vi "readI64.vi"(8 "error in (no error)":errorcluster, 11 "ModbusBuffer in":refnum<class "ModbusBuffer.lvclass">) -> (0 "error out":errorcluster, 2 "Output":i64, 3 "ModbusBuffer out":refnum<class "ModbusBuffer.lvclass">)   [LabVIEW 2016, in "RTModbus.lvlib" / "ModbusBuffer.lvclass"]
uses:
  ModbusBuffer.lvclass
  ModbusBuffer.lvclass/ModbusBuffer.ctl
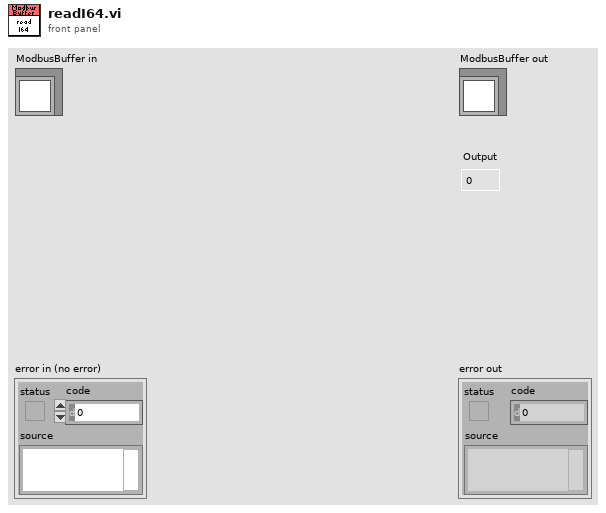
[diagram p1: front panel]
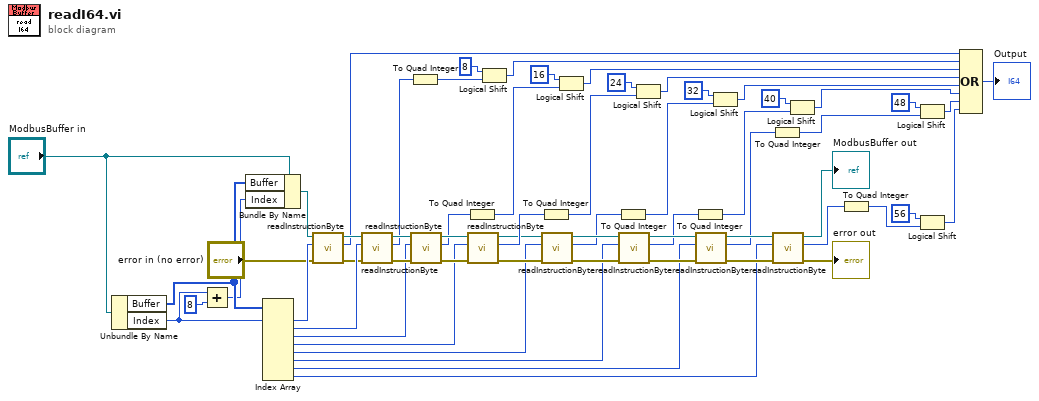
[diagram p0: block diagram]
diagram:
  n1 = Unbundle By Name("ModbusBuffer in") -> ("Buffer"=w60:u16[], "Index"=w56:i32)
  n2 = Add(x=w56, y=8) -> (x+y=w54:i32)
  n3 = Bundle By Name(cluster="ModbusBuffer in", "Buffer"=w60, "Index"=w54) -> (w58:refnum<class "ModbusBuffer.lvclass">)
  n4 = Index Array(array=w60, index #1=w56) -> (element #1=w59:u16, element #2=w52:u16, element #3=w38:u16, element #4=w37:u16, element #5=w12:u16, element #6=w11:u16, element #7=w10:u16, element #8=w9:u16)  [unwired: 7 in]
  n5 = call "readInstructionByte.vi"("error in (no error)"="error in (no error)", "Instruction"=w59, "ModbusBuffer in"=w58) -> ("error out"=w50:errorcluster, "Output"=w51:u8, "ModbusBuffer out"=w53:refnum<class "ModbusBuffer.lvclass">)  [unwired: 6 in]
  n6 = call "readInstructionByte.vi"("error in (no error)"=w50, "Instruction"=w52, "ModbusBuffer in"=w53) -> ("error out"=w44:errorcluster, "Output"=w36:u8, "ModbusBuffer out"=w46:refnum<class "ModbusBuffer.lvclass">)  [unwired: 6 in]
  n7 = To Quad Integer(1:w36) -> (0:w35:i64)
  n8 = call "readInstructionByte.vi"("error in (no error)"=w44, "Instruction"=w38, "ModbusBuffer in"=w46) -> ("error out"=w43:errorcluster, "Output"=w34:u8, "ModbusBuffer out"=w45:refnum<class "ModbusBuffer.lvclass">)  [unwired: 6 in]
  n9 = To Quad Integer(1:w34) -> (0:w33:i64)
  n10 = call "readInstructionByte.vi"("error in (no error)"=w43, "Instruction"=w37, "ModbusBuffer in"=w45) -> ("error out"=w17:errorcluster, "Output"=w32:u8, "ModbusBuffer out"=w22:refnum<class "ModbusBuffer.lvclass">)  [unwired: 6 in]
  n11 = Logical Shift(y=i16 8, x=w35) -> (x << y=w48:i64)
  n12 = To Quad Integer(1:w32) -> (0:w31:i64)
  n13 = call "readInstructionByte.vi"("error in (no error)"=w17, "Instruction"=w12, "ModbusBuffer in"=w22) -> ("error out"=w16:errorcluster, "Output"=w8:u8, "ModbusBuffer out"=w21:refnum<class "ModbusBuffer.lvclass">)  [unwired: 6 in]
  n14 = Logical Shift(y=i16 16, x=w33) -> (x << y=w39:i64)
  n15 = To Quad Integer(1:w8) -> (0:w30:i64)
  n16 = call "readInstructionByte.vi"("error in (no error)"=w16, "Instruction"=w11, "ModbusBuffer in"=w21) -> ("error out"=w15:errorcluster, "Output"=w7:u8, "ModbusBuffer out"=w20:refnum<class "ModbusBuffer.lvclass">)  [unwired: 6 in]
  n17 = Logical Shift(y=i16 24, x=w31) -> (x << y=w40:i64)
  n18 = To Quad Integer(1:w7) -> (0:w27:i64)
  n19 = call "readInstructionByte.vi"("error in (no error)"=w15, "Instruction"=w10, "ModbusBuffer in"=w20) -> ("error out"=w14:errorcluster, "Output"=w6:u8, "ModbusBuffer out"=w19:refnum<class "ModbusBuffer.lvclass">)  [unwired: 6 in]
  n20 = Logical Shift(y=i16 32, x=w30) -> (x << y=w4:i64)
  n21 = To Quad Integer(1:w6) -> (0:w26:i64)
  n22 = call "readInstructionByte.vi"("error in (no error)"=w14, "Instruction"=w9, "ModbusBuffer in"=w19) -> ("error out"=→"error out":errorcluster, "Output"=w5:u8, "ModbusBuffer out"=→"ModbusBuffer out":refnum<class "ModbusBuffer.lvclass">)  [unwired: 6 in]
  n23 = Logical Shift(y=i16 40, x=w27) -> (x << y=w3:i64)
  n24 = To Quad Integer(1:w5) -> (0:w23:i64)
  n25 = Logical Shift(y=i16 48, x=w26) -> (x << y=w2:i64)
  n26 = Logical Shift(y=i16 56, x=w23) -> (x << y=w1:i64)
  n27 = Compound Arithmetic op=OR(w51, w48, w39, w40, w4, w3, w2, w1) -> (→"Output":i64)
